vi "ADC read.vi"() -> (1 "ADC1":i16, 2 "ADC0":i16)   [LabVIEW 2015]
uses:
  <vilib>/Platform/TimedLoop/XDataNode/timing_clust.ctl
  <vilib>/Platform/TimedLoop/XDataNode/nitl_modes.ctl
  <vilib>/Platform/TimedLoop/XDataNode/wakeup.ctl
  <vilib>/rvi/Emulation/niFpgaSctlEmulationGetInTimedLoop.vi
  <vilib>/rvi/Emulation/niFpgaEmulationReportErrorSimple.vi
  <vilib>/rvi/Emulation/niFpgaGetClockAttributes.vi
  <vilib>/rvi/Emulation/niFpgaCriticalErrorInLSC.vi
  <vilib>/rvi/eio/common/nirviEmuTemplateMethod_errors.vi
  <vilib>/Platform/TimedLoop/XDataNode/XDataNode.xnode
  <vilib>/eio/EIONode/EIONode.xnode
  <vilib>/Platform/TimedLoop/XDataNode/XDNodeRunTimeDep.lvlib
panel:
  out "Y P_out0":i16
  out "Y P_out1":i16
  out "Y P_out2":i16
  out "Y P_out3":i16
  out "Y P_out4":i16
  out "Y P_out5":i16
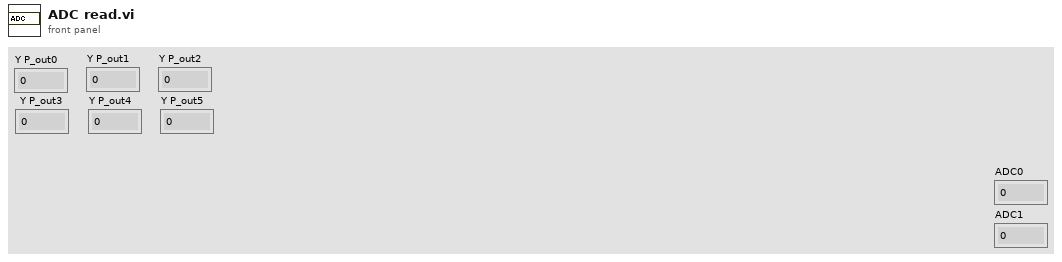
[diagram p1: front panel]
types:
  T1 = typedef "XDNodeRunTimeDep.lvlib/timing_clust.ctl" = cluster{"Expected End [f-1]":u64, "Actual End [f-1]":u64, "Finished Late? [f-1]":bool, "Expected End [i-1]":u64, "Actual End [i-1]":u64, "Finished Late? [i-1]":bool, "Expected Start [i]":u64, "Actual Start [i]":u64, "Expected Start [f]":u64, "Actual Start [f]":u64, "Source Name":string, "Structure Name":string, "Period":i64, "Deadline":i64, "Offset":i64, "Start":i64, "Priority":i32, "Timeout":i32, "Mode":T2, "Wakeup Reason":T3, "Error":errorcluster, "Source Type":string, "Secondary Source Type":string, "Global End Time":u64, "Global Start Time":u64, "Frame Duration":u64, "Iteration Duration":u64, "Assigned CPU":i32, "I/O Scan Engine Mode":u32}
  T2 = typedef "XDNodeRunTimeDep.lvlib/nitl_modes.ctl" = enum32{"No Change", "Process missed periods, maintain original phase", "Discard missed periods, maintain original phase", "Process missed periods, ignore original phase", "Discard missed periods, ignore original phase"}
  T3 = typedef "XDNodeRunTimeDep.lvlib/wakeup.ctl" = enum32{"Normal", "Aborted", "Asynchronous wakeup", "Timing source error", "Timed loop error", "Timeout"}
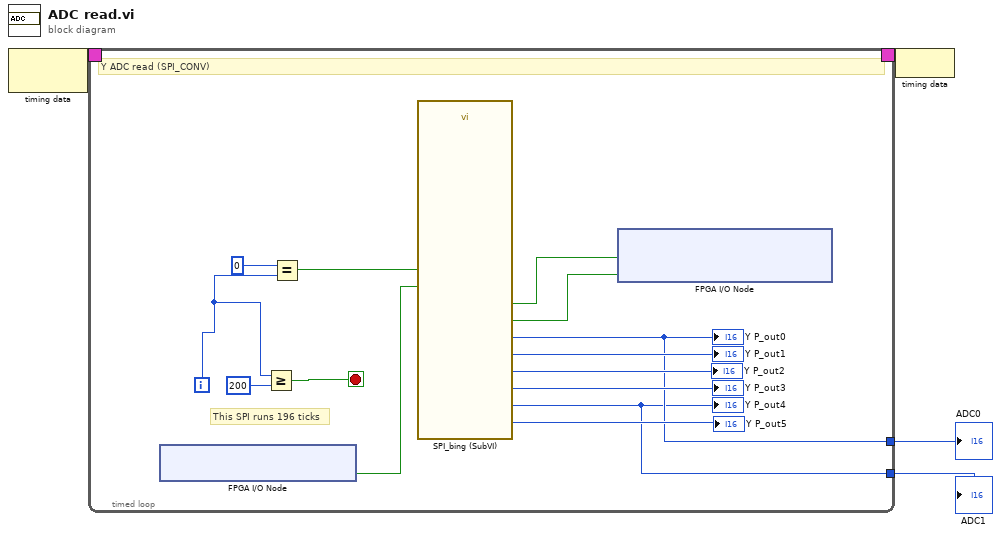
[diagram p0: block diagram]
diagram:
  n1 = node-c288() -> (w4:T1)  [unwired: 1 in]
  n2 = timed-loop "Timed Loop" {
    timing: w4 -> [_]
    timing-out: [_] -> w3
    tunnel: [w7] -> w2
    tunnel: [w6] -> w1
    i -> [w17]
    stop <- w15 stop-if-true
    # "This SPI runs 196 ticks"
    # "Y ADC read (SPI_CONV)"
    n3 = xnode "FPGA I/O Node"() -> ("sbRIO-9651 Socket\\Y_SDO_in"=w12:bool)  [unwired: 1 in, 1 out]
    n4 = Greater Or Equal?(x=w17, y=200) -> (x >= y?=w15:bool)
    n5 = Equal?(x=0, y=w17) -> (x = y?=w14:bool)
    n6 = call "SPI_bing (SubVI).vi"("rst_strb"=w14, "s-data"=w12) -> ("P_out3"=→"Y P_out3":i16, "P_out2"=→"Y P_out2":i16, "SCK"=w13:bool, "P_out1"=→"Y P_out1":i16, "conv"=w5:bool, "P_out5"=→"Y P_out5":i16, "P_out4"=w6:i16, "P_out0"=w7:i16)  [unwired: 4 in, 6 out]
    "Y P_out0" <- w7
    "Y P_out4" <- w6
    n7 = xnode "FPGA I/O Node"("sbRIO-9651 Socket\\Y_SCK_out"=w13, "sbRIO-9651 Socket\\Y_CONV_out"=w5) -> ()  [unwired: 2 in, 2 out]
  }
  "ADC0" <- w2
  "ADC1" <- w1
  n8 = node-c288(w3) -> ()
